vi "ZK注射泵操作.vi"(7 "是否启用通讯通知":bool, 8 "error in (no error)":errorcluster, 9 "注射泵操作步":u16, 10 "注射泵操作":T2, 11 "Slave ID":T1) -> (0 "error out":errorcluster)   [LabVIEW 2016, in "质控单元V2.lvlib"]
uses:
  <vilib>/Plasmionique/MB Master/MB_Master/MB_Master.lvclass
  <vilib>/Plasmionique/MB Master/MB Master.lvlib
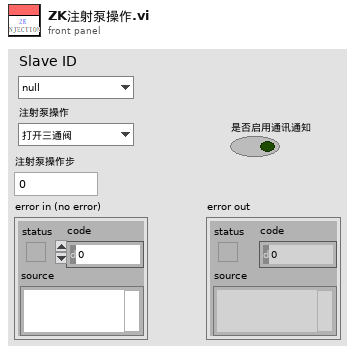
[diagram p1: front panel]
types:
  T1 = typedef "质控单元V2.lvlib/质控slave id.ctl" = enum16{"null", "氨氮", "总磷", "总氮", "CODMn", "CODCr"}
  T2 = typedef "质控单元V2.lvlib/质控注射泵操作.ctl" = enum16{"打开三通阀", "关闭三通阀", "注射泵吸入", "注射泵排出", "注射泵暂停", "注射泵复位"}
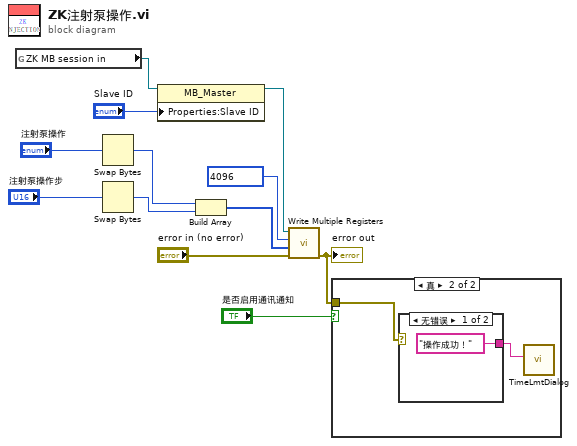
[diagram p0: block diagram]
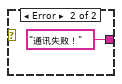
[diagram p3: hidden frame]
diagram:
  n1 = global read "ZK非断电保存全局变量.vi" "ZK MB session in"() -> (w11:refnum<class "MB_Master.lvclass">)
  n2 = Swap Bytes(anything="注射泵操作") -> (byte swapped=w6:u16)
  n3 = Swap Bytes(anything="注射泵操作步") -> (byte swapped=w1:u16)
  n4 = property class="MB_Master"(reference=w11, "Properties:Slave ID"="Slave ID") -> (reference out=w8:refnum<class "MB_Master.lvclass">)  [unwired: 1 in, 1 out]
  n5 = Build Array(w6, w1) -> (w5:u16[])
  n6 = call <vilib>:"Write Multiple Registers.vi"("error in (no error)"="error in (no error)", "values"=w5, "starting address"=u16 4096, "MB session in"=w8) -> ("error out"=w3:errorcluster)  [unwired: 6 in, 1 out]
  "error out" <- w3
  n7 = case shown="真" "是否启用通讯通知" {
    tunnel: w3 -> [_ w14]
    frame False {
    }
    frame True {
      n8 = case shown="无错误" w14 {
        tunnel: ["操作成功！" "通讯失败！"] -> w13
        frame No Error {
        }
        frame Error {
        }
      }
      n9 = call "TimeLmtDialog.vi"("Infoin"=w13) -> ()  [unwired: 11 in]
    }
  }
